vi "Deviation Signal.vi"(2 "Input":dbl[](array[numeric]), 3 "Action":T1) -> (0 "Output":dbl[](array[numeric]))   [LabVIEW 2013]
uses:
  Functional Globals/Action.ctl
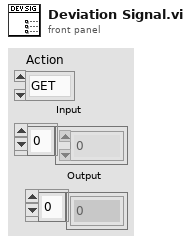
[diagram p1: front panel]
types:
  T1 = typedef "Action.ctl" = enum16{"GET", "PUT", "DELETE"}
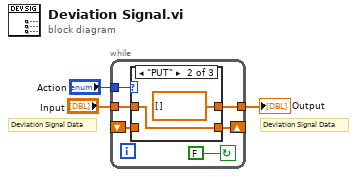
[diagram p0: block diagram]
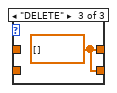
[diagram p3: hidden frame]
diagram:
  # "Deviation Signal Data"
  # "Deviation Signal Data"
  n1 = while {
    tunnel: "Action" -> [w9]
    shift-right: [w7] -> _
    shift-left: _ -> [w5]
    tunnel: "Input" -> [w8]
    tunnel: [w6] -> w1
    stop <- FALSE continue-if-true
    n2 = case shown="\"PUT\"" w9 {
      tunnel: w8 -> [_ w12 _]
      tunnel: [w10 w12 w13] -> w7
      tunnel: [w10 dbl[] [] ("Input") w13] -> w6
      tunnel: w5 -> [w10 _ _]
      frame "GET" {
      }
      frame "PUT" {
      }
      frame "DELETE" {
        w13 = dbl[] [] ("Input")
      }
    }
  }
  "Output" <- w1
